vi "Insert 2D Str Query SQLServer.vi"(7 "Columns":string[](array[string]), 8 "error in (no error)":errorcluster, 9 "Data":string[][](array[string]), 10 "Table":string, 11 "ADODB._Connection":refnum<k7>) -> (0 "error out":errorcluster, 2 "Records Affected":i32, 3 "ADODB._Connection 2":refnum<k7>)   [LabVIEW 2017]
panel:
  out "Query":string
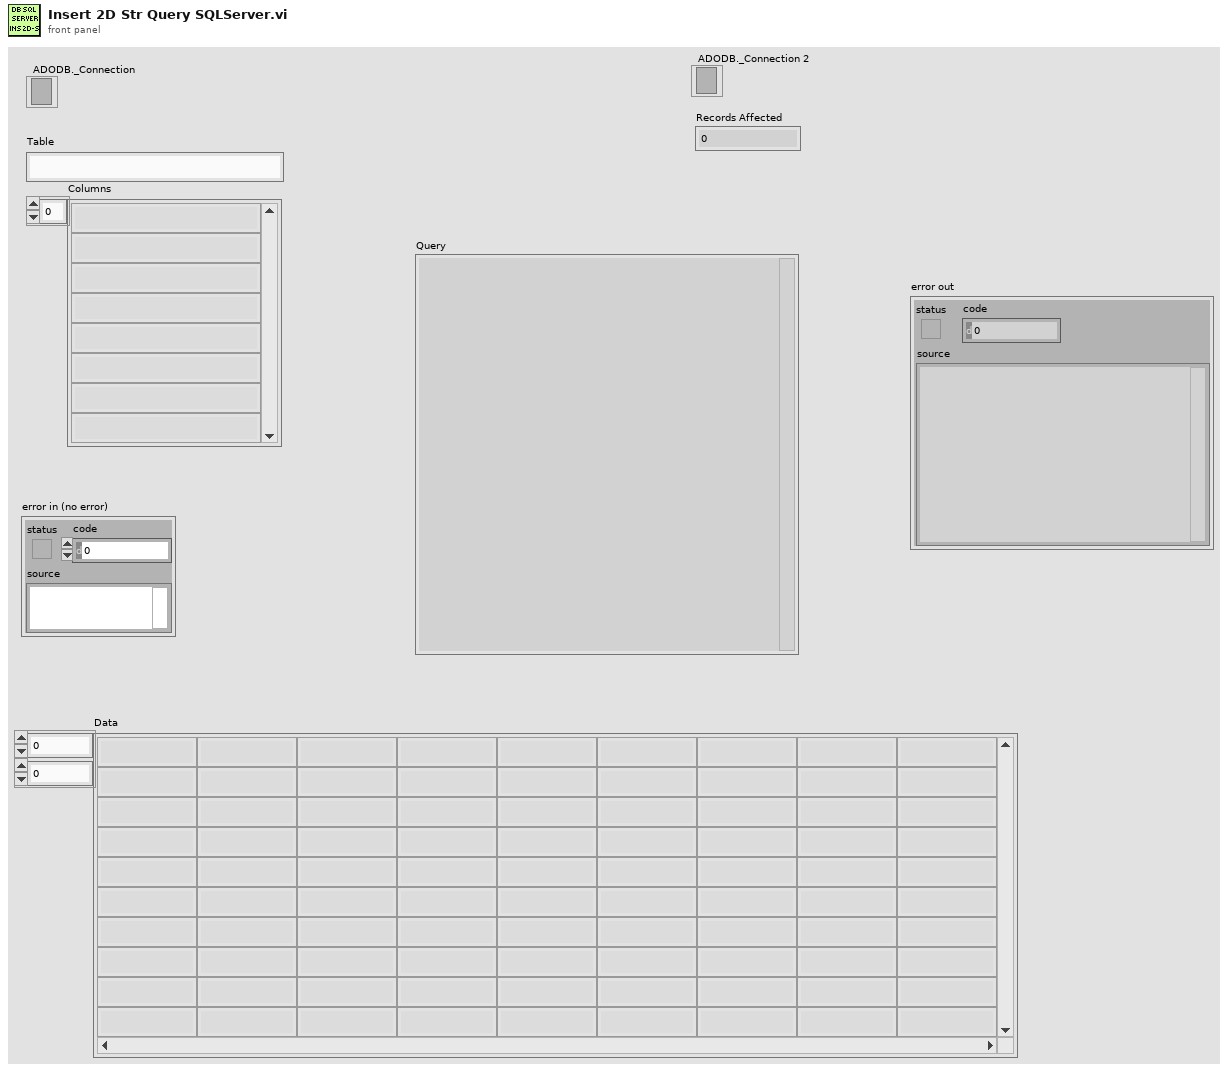
[diagram p1: front panel]
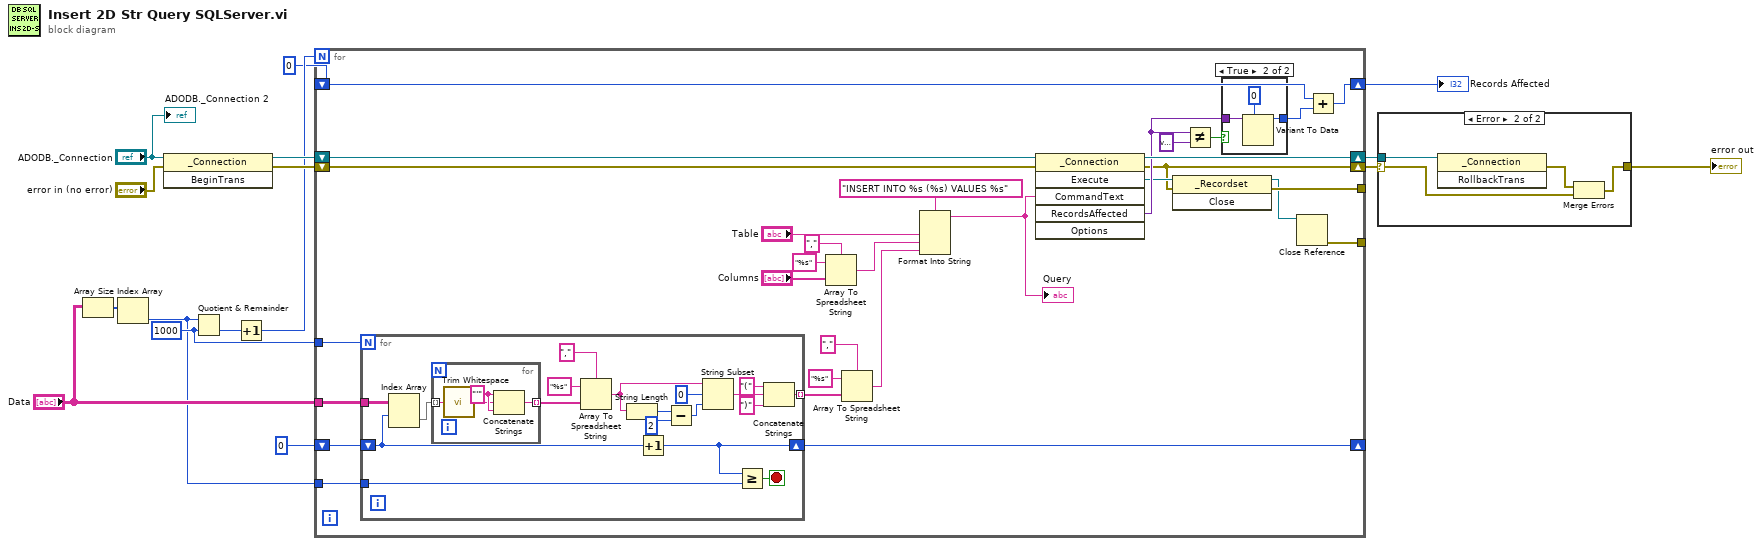
[diagram p0: block diagram]
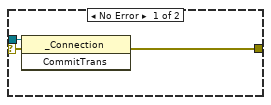
[diagram p3: hidden frame]
diagram:
  w5 = 1000 ("y")
  n1 = Array Size(array="Data") -> (size(s)=w8:i32[])
  n2 = Index Array(array=w8) -> (element=w3:i32)  [unwired: 1 in]
  n3 = invoke class="_Connection" method="BeginTrans"(reference="ADODB._Connection", error in="error in (no error)") -> (reference out=w16:refnum<k7>, error out=w15:errorcluster)  [unwired: 1 in, 1 out]
  n4 = Quotient & Remainder(x=w3, y=w5) -> (floor(x/y)=w7:i32)  [unwired: 1 out]
  n5 = Increment(x=w7) -> (x+1=w6:i32)
  n6 = for {
    N: w6 -> [_]
    tunnel: "Data" -> [w31]
    shift-right: [w19] -> w14
    shift-left: w15 -> [w34]
    shift-right: [w33] -> w13
    shift-left: w16 -> [w36]
    tunnel: w5 -> [w32]
    shift-right: [w29] -> _
    shift-left: 0 ("y") -> [w30]
    tunnel: w3 -> [w28]
    shift-right: [w21] -> w1
    shift-left: 0 ("y") -> [w22]
    tunnel: [w20] -> _
    tunnel: [w17] -> _
    n7 = for {
      N: w32 -> [_]
      tunnel: [w62] -> w38 mode=indexing
      tunnel: w31 -> [w55]
      shift-right: [w52] -> w29
      shift-left: w30 -> [w53]
      tunnel: w28 -> [w51]
      stop <- w50 stop-if-true
      n8 = Index Array(array=w55, index (row)=w53) -> (element=w54:string[])  [unwired: 1 in]
      n9 = for {
        tunnel: w54 -> [w71] mode=indexing
        tunnel: [w69] -> w65 mode=indexing
        w70 = "'" ("string")
        n10 = call <vilib>:"Trim Whitespace.vi"("string"=w71) -> ("trimmed string"=w68:string)  [unwired: 1 in]
        n11 = Concatenate Strings(w70, w68, w70) -> (w69:string)
      }
      n12 = Array To Spreadsheet String(delimiter (Tab)=",", array=w65, 3:"%s" ("format string")) -> (spreadsheet string=w61:string)
      n13 = String Length(string=w61) -> (length=w59:i32)
      n14 = Increment(x=w53) -> (x+1=w52:i32)
      n15 = Subtract(x=w59, y=2) -> (x-y=w56:i32)
      n16 = String Subset(string=w61, offset (0)=0, length (rest)=w56) -> (substring=w57:string)
      n17 = Greater Or Equal?(x=w52, y=w51) -> (x >= y?=w50:bool)
      n18 = Concatenate Strings("(" ("string"), w57, ")" ("string")) -> (w62:string)
    }
    n19 = Array To Spreadsheet String(delimiter (Tab)=",", array="Columns", 3:"%s" ("format string")) -> (spreadsheet string=w41:string)
    n20 = Array To Spreadsheet String(delimiter (Tab)=",", array=w38, 3:"%s" ("format string")) -> (spreadsheet string=w37:string)
    n21 = Format Into String(format string="INSERT INTO %s (%s) VALUES %s", "Table", w41, w37) -> (resulting string=w35:string)  [unwired: 2 in, 1 out]
    "Query" <- w35
    n22 = invoke class="_Connection" method="Execute"(reference=w36, error in=w34, "CommandText"=w35) -> (reference out=w33:refnum<k7>, error out=w19:errorcluster, "Execute"=w24:refnum<k7>, "RecordsAffected"=w27:variant)  [unwired: 3 in, 2 out]
    n23 = invoke class="_Recordset" method="Close"(reference=w24, error in=w19) -> (reference out=w18:refnum<k7>, error out=w20:errorcluster)  [unwired: 1 in, 1 out]
    n24 = Not Equal?(x=w27, y=variant) -> (x != y?=w25:bool)
    n25 = case shown="True" w25 {
      tunnel: [_ w48] -> w23
      tunnel: w27 -> [_ w47]
      frame False {
      }
      frame True {
        n26 = Variant To Data(type=0, Variant=w47) -> (data=w48:i32)  [unwired: 1 in, 1 out]
      }
    }
    n27 = Close Reference(reference=w18) -> (error out=w17:errorcluster)  [unwired: 1 in]
    n28 = Add(x=w22, y=w23) -> (x+y=w21:i32)
  }
  "Records Affected" <- w1
  n29 = case shown="Error" w14 {
    selector: w14 -> [w73 w77]
    tunnel: w13 -> [w74 w78]
    tunnel: [w72 w76] -> w11
    frame No Error {
      n30 = invoke class="_Connection" method="CommitTrans"(reference=w74, error in=w73) -> (error out=w72:errorcluster)  [unwired: 1 in, 2 out]
    }
    frame Error {
      n31 = invoke class="_Connection" method="RollbackTrans"(reference=w78) -> (error out=w75:errorcluster)  [unwired: 2 in, 2 out]
      n32 = Merge Errors(w75, w77) -> (w76:errorcluster)
    }
  }
  "error out" <- w11
  "ADODB._Connection 2" <- "ADODB._Connection"
